vi "Write and Rade(232).vi"(0 "VISA resource name in":refnum<visa-resource-name>="COM2", 1 "write":bool=TRUE, 2 "read":bool=TRUE, 5 "string to write":string="*IDN?\r\n", 7 "ms delay":u32, 9 "baud rate(read)":u32=9600, 11 "error in":errorcluster, 12 "change baud rate(read)":bool) -> (4 "VISA resource name out":refnum<visa-resource-name>, 6 "read string":string, 10 "bytes read":u32, 15 "error out":errorcluster)   [LabVIEW 2009]
uses:
  <vilib>/Instr/_visa.llb/VISA Configure Serial Port (Instr).vi
panel:
  out "error out 2":errorcluster
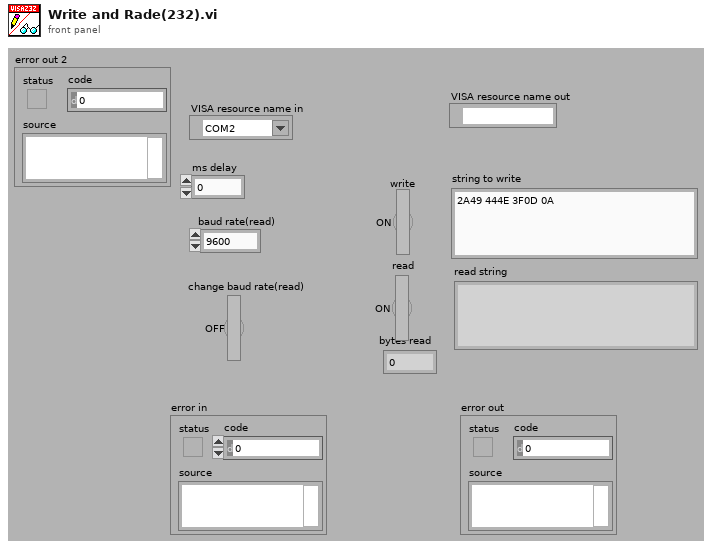
[diagram p1: front panel]
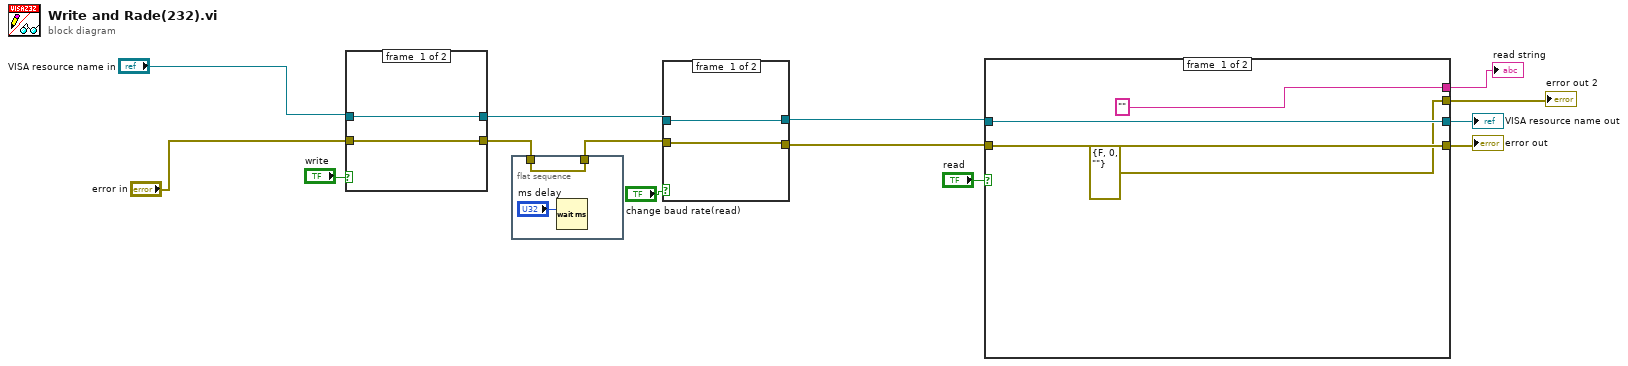
[diagram p0: block diagram]
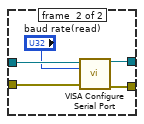
[diagram p2: hidden frame]
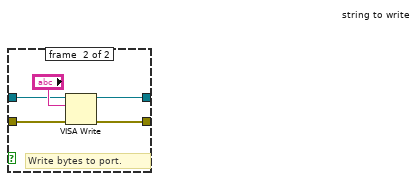
[diagram p3: hidden frame]
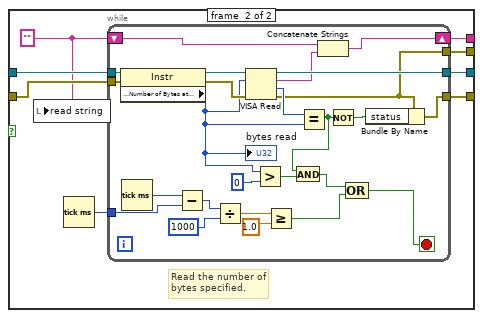
[diagram p4: hidden frame]
diagram:
  n1 = case shown="True" "write" {
    tunnel: [w16 w21] -> w5
    tunnel: "VISA resource name in" -> [w15 w19]
    tunnel: "error in" -> [w16 w18]
    tunnel: [w15 w17] -> w8
    frame #0 {
    }
    frame #1 {
      # "Write bytes to port."
      n2 = VISA Write(VISA resource name=w19, write buffer="string to write", error in (no error)=w18) -> (VISA resource name out=w17:refnum<visa-resource-name>, error out=w21:errorcluster)  [unwired: 1 out]
    }
  }
  n3 = flat-sequence {
    tunnel: [w22] -> w4
    tunnel: w5 -> [w22]
    frame #0 {
      n4 = Wait (ms)(milliseconds to wait="ms delay") -> ()  [unwired: 1 out]
    }
  }
  n5 = case shown="False" "change baud rate(read)" {
    tunnel: w8 -> [w25 w30]
    tunnel: w4 -> [w24 w29]
    tunnel: [w24 w27] -> w3
    tunnel: [w25 w26] -> w10
    frame #0 {
    }
    frame #1 {
      n6 = call-poly "VISA Configure Serial Port"("VISA resource name"=w30, "baud rate (9600)"="baud rate(read)", "error in (no error)"=w29) -> ("VISA resource name out"=w26:refnum<visa-resource-name>, "error out"=w27:errorcluster)  [unwired: 3 in, 8 out]
    }
  }
  n7 = case shown="True" "read" {
    tunnel: w3 -> [w34 w39]
    tunnel: [w34 w42] -> w12
    tunnel: [w33 w41] -> w11
    tunnel: w10 -> [w33 w40]
    tunnel: [errorcluster {"status"=FALSE, "code"=0, "source"=""} ("error out") w37] -> w7
    tunnel: ["" ("read buffer") w36] -> w6
    frame #0 {
    }
    frame #1 {
      w35 = "" ("read buffer")
      # "Read the number of bytes specified."
      n8 = local write "read string"(w35) -> ()
      n9 = Tick Count (ms)() -> (millisecond timer value=w38:u32)
      n10 = while {
        tunnel: [w54] -> w42
        tunnel: [w67] -> w41
        tunnel: w40 -> [w66]
        tunnel: w39 -> [w65]
        tunnel: w38 -> [w56]
        tunnel: [w52] -> w37
        shift-right: [w44] -> w36
        shift-left: w35 -> [w46]
        stop <- w50 stop-if-true
        n11 = property class="Instr"(reference=w66, error in=w65) -> (reference out=w64:refnum<visa-resource-name>, error out=w63:errorcluster, "Serial Settings:Number of Bytes at Serial Port"=w43:u32)
        "bytes read" <- w43
        n12 = Tick Count (ms)() -> (millisecond timer value=w57:u32)
        n13 = Subtract(x=w57, y=w56) -> (x-y=w58:u32)
        n14 = Divide(x=w58, y=u32 1000) -> (x/y=w60:dbl)
        n15 = VISA Read(VISA resource name=w64, byte count=w43, error in (no error)=w63) -> (VISA resource name out=w67:refnum<visa-resource-name>, read buffer=w45:string, return count=w55:u32, error out=w52:errorcluster)
        n16 = Greater?(x=w43, y=u32 0) -> (0:w49:bool)
        n17 = Greater Or Equal?(x=w60, y=1.0) -> (x >= y?=w51:bool)
        n18 = Equal?(x=w55, y=w43) -> (x = y?=w48:bool)
        n19 = And(x=w48, y=w49) -> (x .and. y?=w47:bool)
        n20 = Concatenate Strings(w46, w45) -> (w44:string)
        n21 = Not(x=w48) -> (.not. x?=w53:bool)
        n22 = Compound Arithmetic op=OR(w47, w51) -> (w50:bool)
        n23 = Bundle By Name(cluster=w52, "status"=w53) -> (w54:errorcluster)
      }
    }
  }
  "error out" <- w12
  "VISA resource name out" <- w11
  "error out 2" <- w7
  "read string" <- w6
